vi "GetFPGA.vi"(11 "Device in":refnum<class "Device.lvclass">) -> (2 "FPGA API.lvclass":refnum<class "FPGA API.lvclass">)   [LabVIEW 2019, in "Device.lvclass"]
uses:
  Device.lvclass
  FPGA_API_class/FPGA API.lvclass
  Device.lvclass/Device.ctl
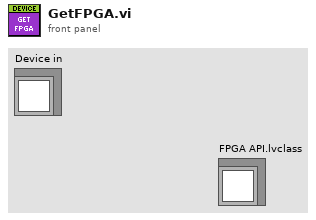
[diagram p1: front panel]
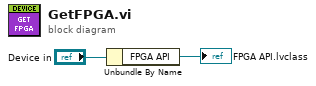
[diagram p0: block diagram]
diagram:
  n1 = Unbundle By Name("Device in") -> ("FPGA API"=→"FPGA API.lvclass":refnum<class "FPGA API.lvclass">)
